vi "Subvi buffer.vi"(0 "Cluster in":cluster{"FIFO name":refnum<k21>, "timeout":i32}={"FIFO name"="FIFO", "timeout"=0}, 8 "Buffer name":refnum<k21>="AO0 buffer") -> ()   [LabVIEW 2017]
uses:
  <vilib>/rvi/DataTransferAndStorage/Container/Common/niFpgaContainerExecOnDevCompGetState.vi
  <vilib>/rvi/Emulation/niFpgaEmulationIsFPGAContextNoSignature.vi
  <vilib>/rvi/Emulation/niFpgaSctlEmulationGetInTimedLoop.vi
  <vilib>/rvi/errors/niFpgaSetErrorForExecOnDevCompSimple.vi
  <vilib>/rvi/eio/common/nirviEmuReportErrorAndStop.vi
  <vilib>/rvi/DataTransferAndStorage/Container/Common/niFpgaContainerGetUniqueNameForEmu.vi
  <vilib>/rvi/FIFO/Fifo_Resource/nirvififoEmulationSetSize.vi
  <vilib>/rvi/FIFO/Fifo_Resource/nirviFifoEmulationQueueMgr.vi
  <instcachedir>/0/nirviFifoEmulationQueueMgr_E5CAEC123FF24DC58D834DCA3CDAA9B5.lvgen/nirviFifoEmulationQueueMgr_E5CAEC123FF24DC58D834DCA3CDAA9B5_001.vi
  <vilib>/rvi/FIFO/Fifo_Resource/nirvififoEmulationDetermineInputValidOut.vi
  <vilib>/rvi/FIFO/Fifo_Resource/nirvififoEmulationCreateLock.vi
  <vilib>/rvi/Emulation/niFpgaProcessEmulError.vi
  <vilib>/rvi/FIFO/Fifo_Resource/nirvififoEmulationObtainLock.vi
  <vilib>/rvi/FIFO/Fifo_Resource/nirvififoEmulationReleaseLock.vi
  <vilib>/rvi/occurrence/nirviWaitOnOccurrenceBase.vi
  <vilib>/rvi/errors/nirviReportUnexpectedCaseInternalError.vi
  <vilib>/rvi/errors/nirviReportUnexpectedCaseInternalError (U32).vi
  <vilib>/Utility/error.llb/Clear Errors.vi
  <vilib>/rvi/interface/RandomDataEmulation/niFpgaRandomDataHandleErrors.vi
  <vilib>/rvi/Memory/Memory_Emulation/niFpgaMemoryEmulationCacheClearOnFirstRun.vi
  <vilib>/rvi/Memory/Memory_Emulation/nirvimemoryEmulationManagerCache_MakeExclusive.vi
  <vilib>/rvi/Memory/Memory_Emulation/niFpgaMemoryEmulationValidateCache.vi
  <vilib>/rvi/Memory/Memory_Emulation/nirvimemoryEmulationManagerCache_InsertValue.vi
  <vilib>/rvi/Memory/Memory_Emulation/nirvimemoryEmulationManagerCache_ReleaseExclusive.vi
  <vilib>/rvi/Memory/Memory_Emulation/nirvimemoryEmulationManagerCache_GetValue.vi
  <vilib>/rvi/Memory/Memory_Emulation/nirvimemoryEmulationManagerCache_SetValue.vi
  <vilib>/rvi/Emulation/niFpgaSctlEmulationResourceMgr.vi
  <vilib>/rvi/DataTransferAndStorage/Container/XNode/niFpgaContainer.xnode
  <vilib>/rvi/FIFO/Fifo_Resource/niFpgaFifoEmulationRefIn.vi
  <vilib>/rvi/Memory/Memory_Emulation/niFpgaMemoryEmulationRefIn.vi
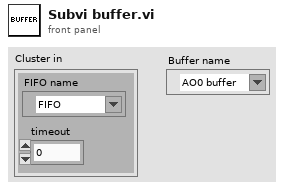
[diagram p1: front panel]
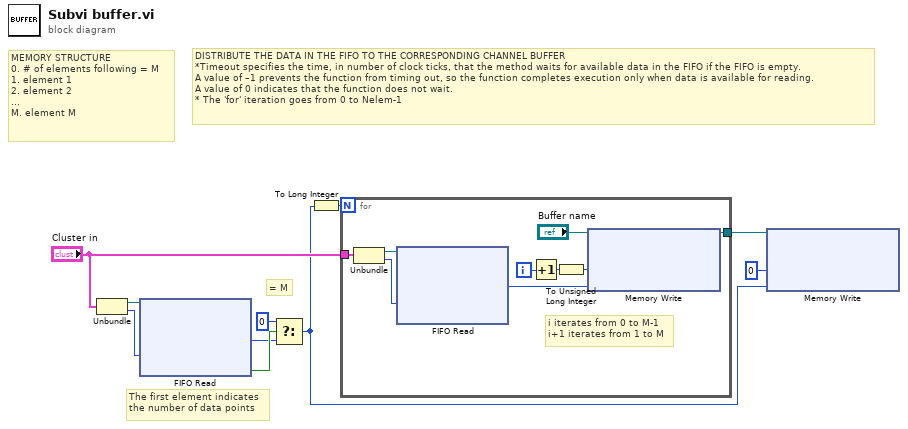
[diagram p0: block diagram]
diagram:
  # "= M"
  # "MEMORY STRUCTURE\n0. # of elements following = M\n1. element 1\n2. element 2\n...\nM. element M"
  # "The first element indicates\nthe number of data points"
  # "DISTRIBUTE THE DATA IN THE FIFO TO THE CORRESPONDING CHANNEL BUFFER\n*Timeout specifies the time, in number of clock ticks, that the method waits for available data in the FIFO if the FIFO is empty.\nA value of –1 prevents the function from timing out, so the function completes execution only when data is available for reading.\nA value of 0 indicates that the function does not wait.\n* The 'for' iteration goes from 0 to Nelem-1"
  n1 = Unbundle("Cluster in") -> ("FIFO name"=w10:refnum<k21>, "timeout"=w9:i32)
  n2 = xnode ("FIFO Read")("Timeout"=w9, "FIFO In"=w10) -> ("Element"=w7:u32, "Timed Out?"=w8:bool)  [unwired: 1 out]
  n3 = Select(t=u32 0, s=w8, f=w7) -> (s? t:f=w1:u32)
  n4 = To Long Integer(number=w1) -> (32bit integer=w2:i32)
  n5 = for {
    N: w2 -> [_]
    tunnel: "Cluster in" -> [w18]
    tunnel: [w12] -> w4
    i -> [w14]
    # "i iterates from 0 to M-1\ni+1 iterates from 1 to M"
    n6 = Unbundle(w18) -> ("FIFO name"=w17:refnum<k21>, "timeout"=w13:i32)
    n7 = xnode ("FIFO Read")("FIFO In"=w17, "Timeout"=w13) -> ("Element"=w19:u32)  [unwired: 2 out]
    n8 = Increment(x=w14) -> (x+1=w15:i32)
    n9 = To Unsigned Long Integer(number=w15) -> (unsigned 32bit integer=w11:u32)
    n10 = xnode ("Memory Write")("Memory In"="Buffer name", "Address"=w11, "Data"=w19) -> ("Memory Out"=w12:refnum<k21>)
  }
  n11 = xnode ("Memory Write")("Address"=u32 0, "Data"=w1, "Memory In"=w4) -> ()  [unwired: 1 out]
